vi "Color String.vi"(7 "Options":T1, 8 "error in (no error)":errorcluster, 9 "Config.List":string[](array[string]), 10 "String.Value":string, 11 "String":refnum<vi>) -> (0 "error out":errorcluster)   [LabVIEW 2021, in "Autocomplete Textbox.lvlib"]
uses:
  Autocomplete Textbox.lvlib
  Color String Options.ctl
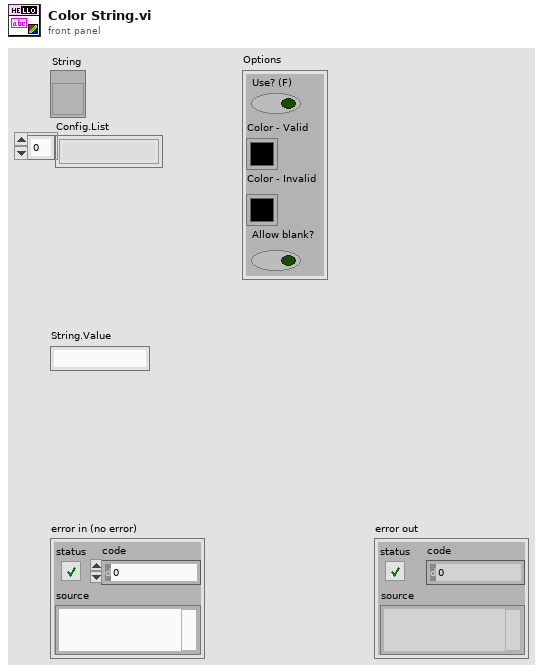
[diagram p1: front panel]
types:
  T1 = typedef "Autocomplete Textbox.lvlib/Color String Options.ctl" = cluster{"Use? (F)":bool, "Color - Valid":u32, "Color - Invalid":u32, "Allow blank?":bool}
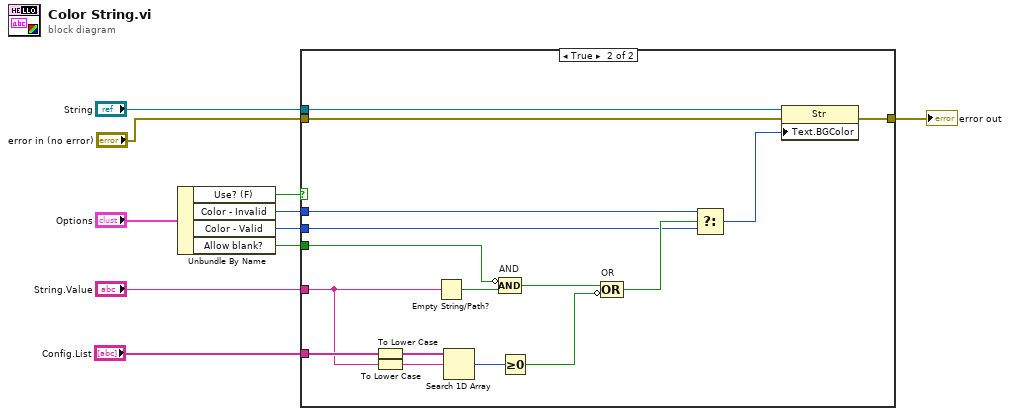
[diagram p0: block diagram]
diagram:
  n1 = Unbundle By Name("Options") -> ("Use? (F)"=w2:bool, "Color - Invalid"=w6:u32, "Color - Valid"=w5:u32, "Allow blank?"=w7:bool)
  n2 = case shown="True" w2 {
    tunnel: "String" -> [_ w27]
    tunnel: "String.Value" -> [_ w12]
    tunnel: w7 -> [_ w25]
    tunnel: w6 -> [_ w22]
    tunnel: w5 -> [_ w21]
    tunnel: "error in (no error)" -> [w11 w19]
    tunnel: [w11 w18] -> w3
    tunnel: "Config.List" -> [_ w15]
    frame False {
    }
    frame True {
      n3 = To Lower Case(string=w15) -> (all lower case string=w14:string[])
      n4 = To Lower Case(string=w12) -> (all lower case string=w13:string)
      n5 = Empty String/Path?(string/path=w12) -> (empty?=w26:bool)
      n6 = Search 1D Array(1D array=w14, element=w13) -> (index of element=w17:i32)  [unwired: 1 in]
      n7 = Compound Arithmetic op=AND "AND"(invert w25, w26) -> (w24:bool)
      n8 = Greater Or Equal To 0?(x=w17) -> (x >= 0?=w16:bool)
      n9 = Compound Arithmetic op=OR "OR"(w24, invert w16) -> (w23:bool)
      n10 = Select(t=w22, s=w23, f=w21) -> (s? t:f=w20:u32)
      n11 = property class="Str"(reference=w27, error in=w19, "Text.BGColor"=w20) -> (error out=w18:errorcluster)  [unwired: 1 out]
    }
  }
  "error out" <- w3
